vi "Lookup API.vi"(7 "API Type":refnum<class "API.lvclass">, 8 "error in (no error)":errorcluster, 10 "Identity":refnum<class "Identity.lvclass">, 11 "VolatusAPI in":refnum<class "VolatusAPI.lvclass">) -> (0 "error out":errorcluster, 2 "API":refnum<class "API.lvclass">, 3 "VolatusAPI out":refnum<class "VolatusAPI.lvclass">)   [LabVIEW 2020, in "Volatus.lvlib" / "VolatusAPI.lvclass"]
uses:
  VolatusAPI.lvclass
  VolatusAPI.lvclass/VolatusAPI.ctl
  Identity/Identity.lvclass
  API/API.lvclass
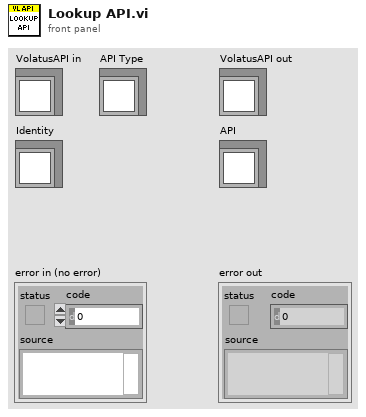
[diagram p1: front panel]
types:
  T1 = typedef "Volatus.lvlib/VolatusAPI.lvclass/APIs Ref.ctl" = cluster{"API Numbers":map{string, u32}, "APIs":map{u32, refnum<class "API.lvclass">}, "Next API":u32}
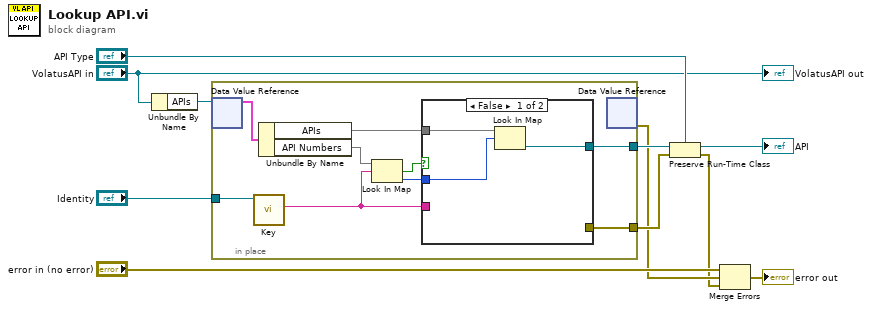
[diagram p0: block diagram]
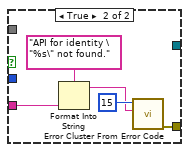
[diagram p2: hidden frame]
diagram:
  n1 = Unbundle By Name("VolatusAPI in") -> ("APIs"=w3:refnum<data-value>)
  n2 = in-place {
    in-place-border: "Identity" -> [w20]
    in-place-border: [w14] -> w6
    in-place-border: [w13] -> w5
    n3 = in-place-dvr #1(w3) -> (w12:T1)  [unwired: 1 out]
    n4 = call "Key.vi"("Identity in"=w20) -> ("Key"=w15:string)  [unwired: 10 in]
    n5 = Unbundle By Name(w12) -> ("APIs"=w17:map{u32, refnum<class "API.lvclass">}, "API Numbers"=w19:map{string, u32})
    n6 = Look In Map(map=w19, key=w15) -> (key not found?=w18:bool, value=w16:u32)  [unwired: 1 in]
    n7 = case shown="False" w18 {
      tunnel: w17 -> [w23 _]
      tunnel: w16 -> [w22 _]
      tunnel: w15 -> [_ w27]
      tunnel: [w21 _] -> w14
      tunnel: [_ w24] -> w13
      frame False {
        n8 = Look In Map(map=w23, key=w22) -> (value=w21:refnum<class "API.lvclass">)  [unwired: 1 in, 1 out]
      }
      frame True {
        n9 = Format Into String(format string="API for identity \"%s\" not found.", w27) -> (resulting string=w25:string)  [unwired: 2 in, 1 out]
        n10 = call <vilib>:"Error Cluster From Error Code.vi"("error message (\"\")"=w25, "error code (0)"=15) -> ("error out"=w24:errorcluster)  [unwired: 7 in]
      }
    }
    n11 = in-place-dvr #1() -> (w2:errorcluster)  [unwired: 1 in, 1 out]
  }
  n12 = Preserve Run-Time Class(object in=w6, error in=w5, 2:"API Type") -> (object out=→"API":refnum<class "API.lvclass">, error out=w1:errorcluster)
  n13 = Merge Errors("error in (no error)", w2, w1) -> (→"error out":errorcluster)
  "VolatusAPI out" <- "VolatusAPI in"
